vi "Create Array (1D).vi"() -> ()   [LabVIEW 2019]
panel:
  in  "My Numeric Array":dbl[](array[numeric])=[5.0, 10.0, 15.0, 20.0, 25.0]
  out "Waveform Graph":dbl[](graph)
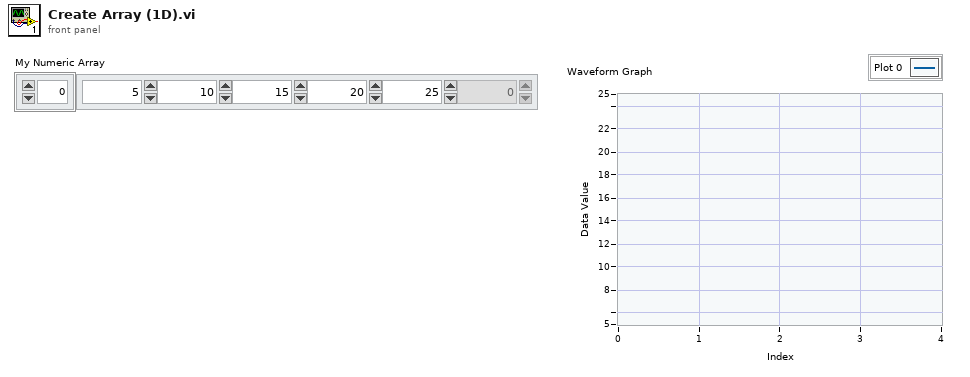
[diagram p1: front panel]
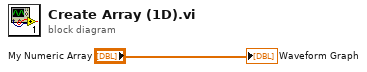
[diagram p0: block diagram]
diagram:
  "Waveform Graph" <- "My Numeric Array"
